vi "LabVIEW Data Type to Measurement Data Type.vi"(8 "error in":errorcluster, 11 "variant":variant) -> (0 "error out":errorcluster, 1 "supported?":bool, 2 "array?":bool, 3 "grpc type":T1, 4 "message type":string, 5 "name":string)   [LabVIEW 2020, in "Measurement Plugin Measurement Server.lvlib"]
uses:
  Measurement Plugin Measurement Server.lvlib
  TypeDefs/Google Protobuf Field Kind.ctl
  <vilib>/Utility/Data Type/NI_Data Type.lvlib
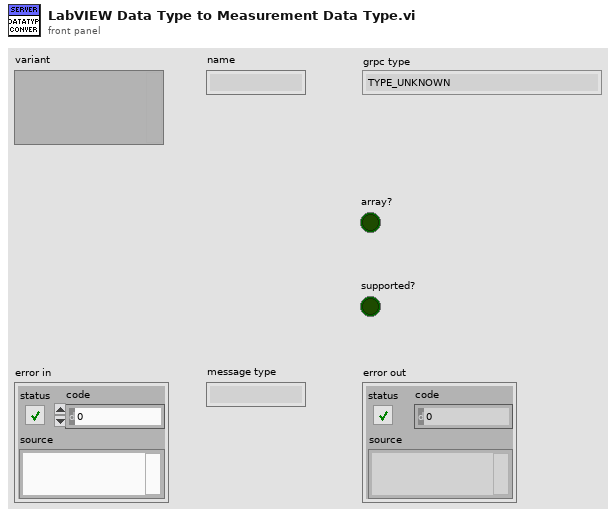
[diagram p1: front panel]
types:
  T1 = typedef "Measurement Plugin Measurement Server.lvlib/Google Protobuf Field Kind.ctl" = enum32{"TYPE_UNKNOWN", "TYPE_DOUBLE", "TYPE_FLOAT", "TYPE_INT64", "TYPE_UINT64", "TYPE_INT32", "TYPE_FIXED64", "TYPE_FIXED32", "TYPE_BOOL", "TYPE_STRING", "TYPE_GROUP", "TYPE_MESSAGE", "TYPE_BYTES", "TYPE_UINT32", "TYPE_ENUM", "TYPE_SFIXED32", "TYPE_SFIXED64", "TYPE_SINT32", "TYPE_SINT64"}
  T2 = typedef "NI_Data Type.lvlib/Data Type.ctl" = enum8{"Invalid Type", "Void", "I8", "I16", "I32", "I64", "U8", "U16", "U32", "U64", "Single Float", "Double Float", "Extended Float", "Single Complex", "Double Complex", "Extended Complex", "Enum U8", "Enum U16", "Enum U32", "Enum U64", "Single Float With Unit", "Double Float With Unit", "Extended Float With Unit", "Single Complex with Unit", "Double Complex with Unit", "Extended Complex with Unit", "Boolean", "String", "Path", "Picture", "Tag", "Array", "Cluster", "Variant", "LV Variant", "Waveform", "Timestamp", "Digital Waveform", "Digital Data", "ExpressData", "Refnum", "External Data", "VI", "Poly VI", "LabVIEW Class Instance", "Fixed Point", "Set Collection", "Map Collection"}
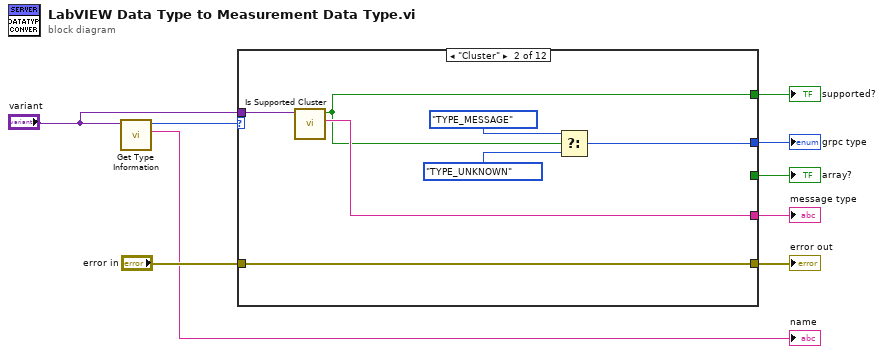
[diagram p0: block diagram]
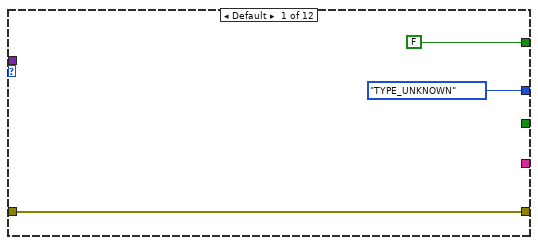
[diagram p2: hidden frame]
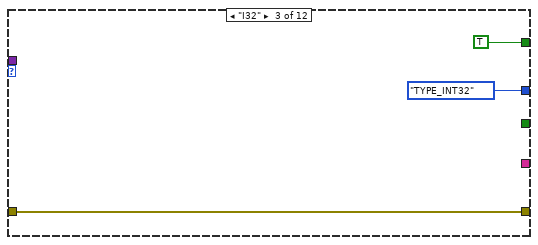
[diagram p3: hidden frame]
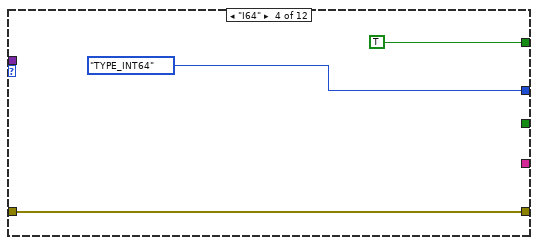
[diagram p4: hidden frame]
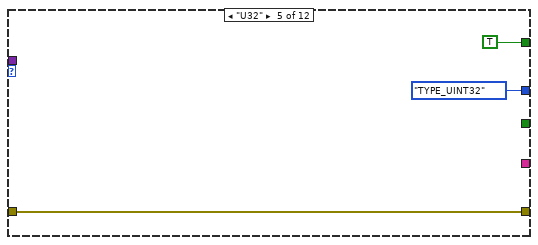
[diagram p5: hidden frame]
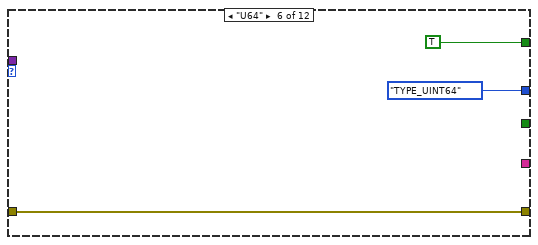
[diagram p6: hidden frame]
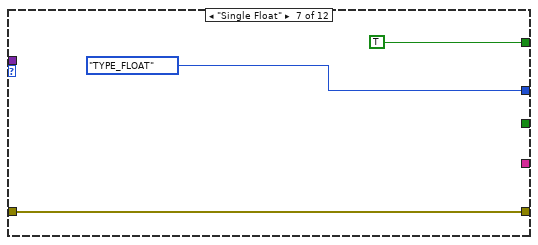
[diagram p7: hidden frame]
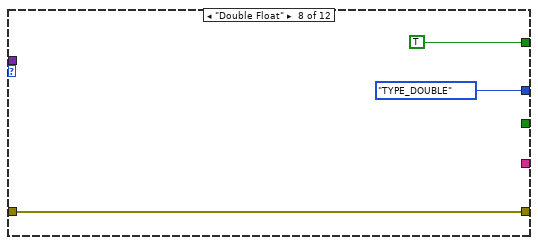
[diagram p8: hidden frame]
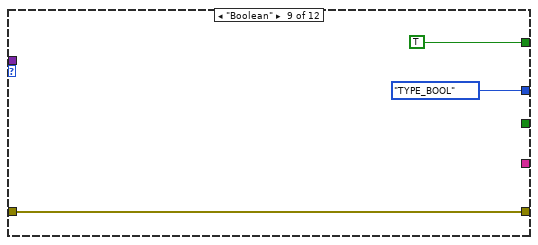
[diagram p9: hidden frame]
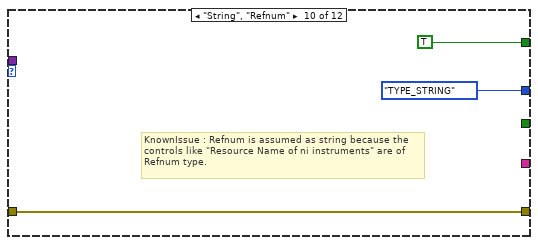
[diagram p10: hidden frame]
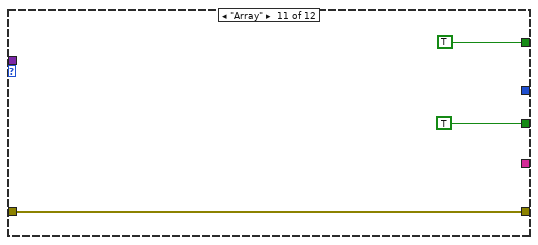
[diagram p11: hidden frame]
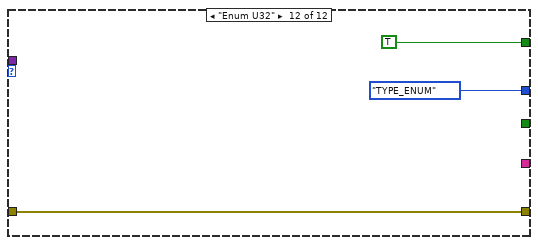
[diagram p12: hidden frame]
diagram:
  n1 = call <vilib>:"Get Type Information.vi"("variant"="variant") -> ("name"=→"name":string, "type"=w4:T2)  [unwired: 6 in, 3 out]
  n2 = case shown="\"Cluster\"" w4 {
    tunnel: [Google_Protobuf_Field_Kind."TYPE_UNKNOWN" ("MessageElementType") w14 Google_Protobuf_Field_Kind."TYPE_INT32" ("MessageElementType") Google_Protobuf_Field_Kind."TYPE_INT64" ("MessageElementType") Google_Protobuf_Field_Kind."TYPE_UINT32" ("MessageElementType") Google_Protobuf_Field_Kind."TYPE_UINT64" ("MessageElementType") Google_Protobuf_Field_Kind."TYPE_FLOAT" ("MessageElementType") Google_Protobuf_Field_Kind."TYPE_DOUBLE" ("MessageElementType") Google_Protobuf_Field_Kind."TYPE_BOOL" ("MessageElementType") Google_Protobuf_Field_Kind."TYPE_STRING" ("MessageElementType") _ Google_Protobuf_Field_Kind."TYPE_ENUM" ("MessageElementType")] -> w9
    tunnel: [FALSE w13 TRUE TRUE TRUE TRUE TRUE TRUE TRUE TRUE TRUE TRUE] -> w8
    tunnel: [_ _ _ _ _ _ _ _ _ _ TRUE _] -> w7
    tunnel: "error in" -> [w10 w19 w20 w23 w26 w29 w32 w35 w38 w41 w44 w49]
    tunnel: [w10 w19 w20 w23 w26 w29 w32 w35 w38 w41 w44 w49] -> w5
    tunnel: "variant" -> [_ w18 _ _ _ _ _ _ _ _ _ _]
    tunnel: [_ w17 _ _ _ _ _ _ _ _ _ _] -> w2
    frame Default {
    }
    frame "Cluster" {
      n3 = call "Is Supported Cluster.vi"("variant"=w18) -> ("message type"=w17:string, "supported?"=w13:bool)  [unwired: 9 in]
      n4 = Select(t=Google_Protobuf_Field_Kind."TYPE_MESSAGE" ("MessageElementType"), s=w13, f=Google_Protobuf_Field_Kind."TYPE_UNKNOWN" ("MessageElementType")) -> (s? t:f=w14:T1)
    }
    frame "I32" {
    }
    frame "I64" {
    }
    frame "U32" {
    }
    frame "U64" {
    }
    frame "Single Float" {
    }
    frame "Double Float" {
    }
    frame "Boolean" {
    }
    frame "String", "Refnum" {
      # "KnownIssue : Refnum is assumed as string because the controls like \"Resource Name of ni instruments\" are of Refnum type."
    }
    frame "Array" {
    }
    frame "Enum U32" {
    }
  }
  "grpc type" <- w9
  "supported?" <- w8
  "array?" <- w7
  "error out" <- w5
  "message type" <- w2
